vi "SnapColorImage.vi"(3 "error in (no error)":errorcluster, 5 "QT Ref In":T1) -> (0 "error out":errorcluster={"status"=TRUE, "code"=-43, "source"=""}, 1 "Image Out":T2 {"Dialogs" format="%.0b"}, 2 "QT Ref Out":T1)   [LabVIEW 2024]
doc: "This VI takes a 24 bit color image from a live camera. The 24 bit image consists of three channels, each at 8 bit (red, green, and blue)."
uses:
  <userlib>/ImageProcessing/QTLIB_2595_LV86/QT_Ref.ctl
  <userlib>/ImageProcessing/QTLIB_2595_LV86/QT_Image.ctl
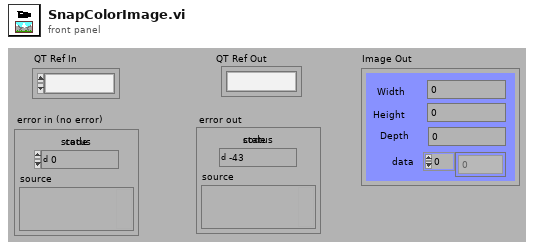
[diagram p1: front panel]
types:
  T1 = typedef "QT_Ref.ctl" = refnum<k1>
  T2 = typedef "QT_Image.ctl" = cluster{"Width":i32, "Height":i32, "Depth":i32, "data":u8[], "Compressed data":u8[], "Color table":u32[], "Duration":i32, "Options":i32, "Timestamp":i32, "ID":i32, "Reserved":i32, "Dialogs":u32}
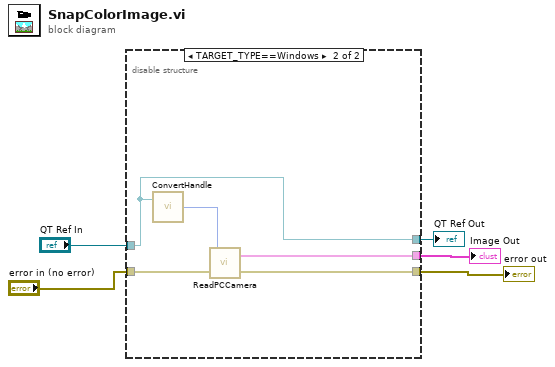
[diagram p0: block diagram]
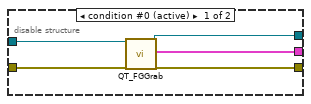
[diagram p2: hidden frame]
diagram:
  n1 = disable-structure shown="TARGET_TYPE==Windows" {
    disable-tunnel: "QT Ref In" -> [w10 w14]
    disable-tunnel: "error in (no error)" -> [w9 w13]
    disable-tunnel: [w8 w15] -> w3
    disable-tunnel: [w7 w12] -> w2
    disable-tunnel: [w6 w14] -> w1
    frame condition #0 (active) {
      n2 = call <userlib>:"QT_FGGrab.vi"("QT Ref In"=w10, "error in (no error)"=w9) -> ("QT Ref Out"=w6:T1, "Image/Movie Out"=w7:T2, "error out"=w8:errorcluster)  [unwired: 4 in, 11 out]
    }
    frame condition #1 {
      n3 = call <vilib>:"ConvertHandle.vi"("QT Ref In"=w14) -> ("Camera Reference"=w11:i64)  [unwired: 1 in, 1 out]
      n4 = call <vilib>:"ReadPCCamera.vi"("error in (no error)"=w13, "Camera Reference"=w11) -> ("error out"=w15:errorcluster, "PC Image Out"=w12:T2)
    }
  }
  "error out" <- w3
  "Image Out" <- w2
  "QT Ref Out" <- w1
